vi "main.vi"() -> ()   [LabVIEW 2015]
uses:
  Type Definitions/Tabs.ctl
  Type Definitions/Technique_selector(Combo box).ctl
  Type Definitions/UI_States.ctl
  Type Definitions/UI_Data.ctl
  support VIs/Message Queue/Enqueue Message (Single).vi
  <vilib>/Utility/error.llb/Error Cluster From Error Code.vi
  <vilib>/ErrorRing/Error Ring.xnode
  support VIs/User Event - Stop/User Event - Stop.lvlib
  support VIs/Message Queue/Message Queue.lvlib
  Techniques/CV/CV.lvlib
panel:
  in  "Combo Box":T1
  in  "Tabs":T2
  out "Cluster 2":T3
  in  "Error In":errorcluster
  in  "Preferences Button":bool
  in  "Settings Button":bool
  in  "File Path Control":path
  in  "Play Button":bool
  in  "Record Button":bool
  in  "Process Stop Button":bool
  in  "Stop Button":bool
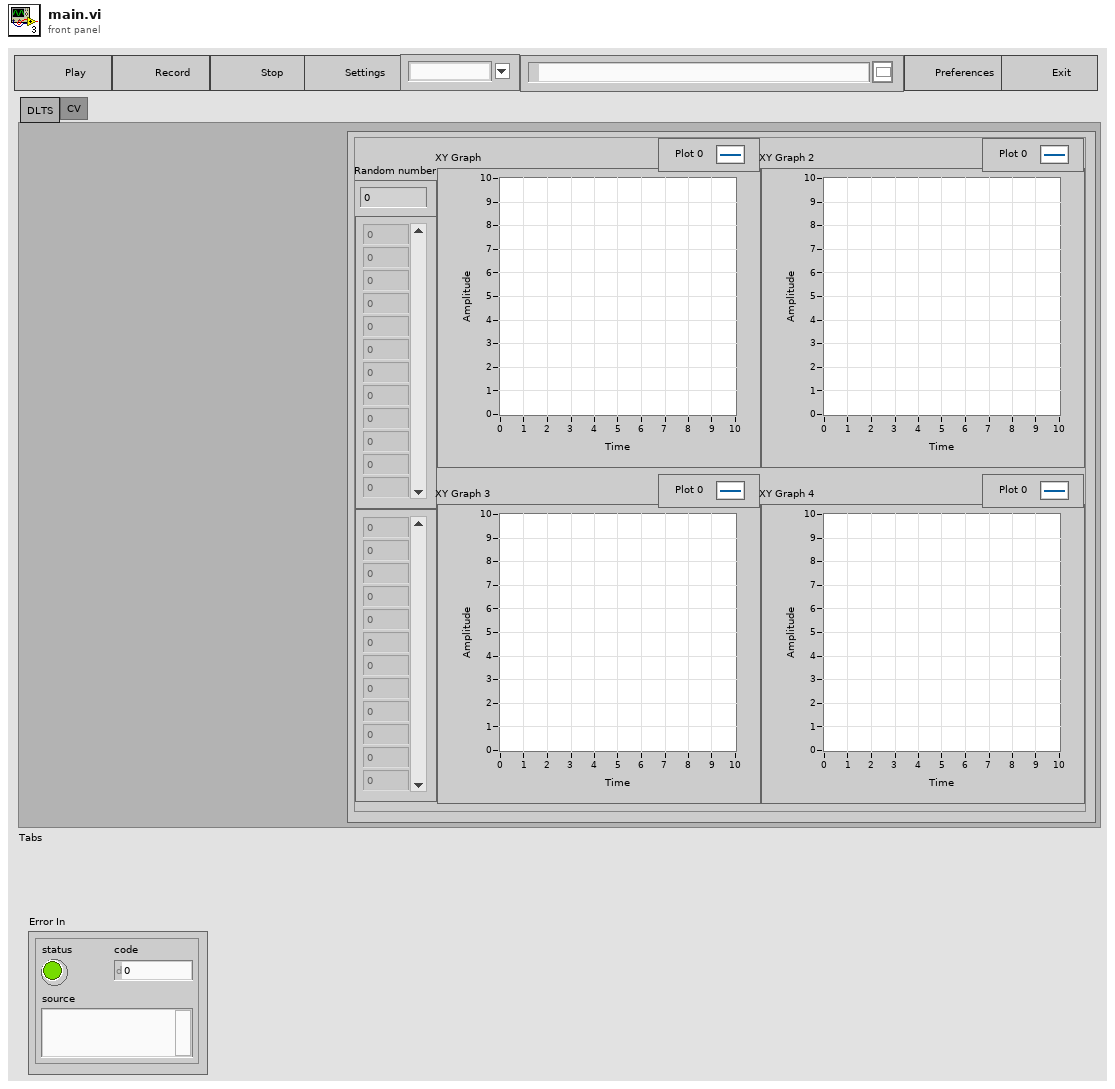
[diagram p1: front panel]
types:
  T1 = typedef "Technique_selector(Combo box).ctl" = string
  T2 = typedef "Tabs.ctl" = enum32{"DLTS", "CV"}
  T3 = cluster{"Array - Numeric 2":dbl[], "XY Graph":cluster{"X":dbl, "Y":dbl}[], "XY Graph 2":cluster{"X":dbl, "Y":dbl}[], "XY Graph 3":cluster{"X":dbl, "Y":dbl}[], "XY Graph 4":cluster{"X":dbl, "Y":dbl}[], "Array - Numeric":dbl[], "Random number":dbl}
  T4 = typedef "UI_Data.ctl" = cluster{"Play Button":refnum<vi>, "Record Button":refnum<vi>, "Stop Button":refnum<vi>, "Settings Button":refnum<vi>, "Preferences Button":refnum<vi>, "Exit Button":refnum<vi>, "Technique Enum":refnum<vi>, "File Path":refnum<vi>}
  T5 = typedef "UI_States.ctl" = enum16{"Idle", "Acquiring and Logging", "Waiting for Exit", "Waiting for Exit (Acq Stoppet)", "Waiting for Exit (Log Stoppet)", "Waiting for Stop", "Waiting for Stop (Acq Stoppet)", "Waiting for Stop (Log Stoppet)"}
  T6 = typedef "Message Queue.lvlib/All Message Queues.ctl" = cluster{"UI":refnum<queue>, "CV Acquisition":refnum<queue>, "CV Logging":refnum<queue>, "IV Acquisition":refnum<queue>, "IV Logging":refnum<queue>, "DLTS Acquisiton":refnum<queue>, "DLTS Logging":refnum<queue>, "Acquisition":refnum<queue>, "Logging":refnum<queue>}
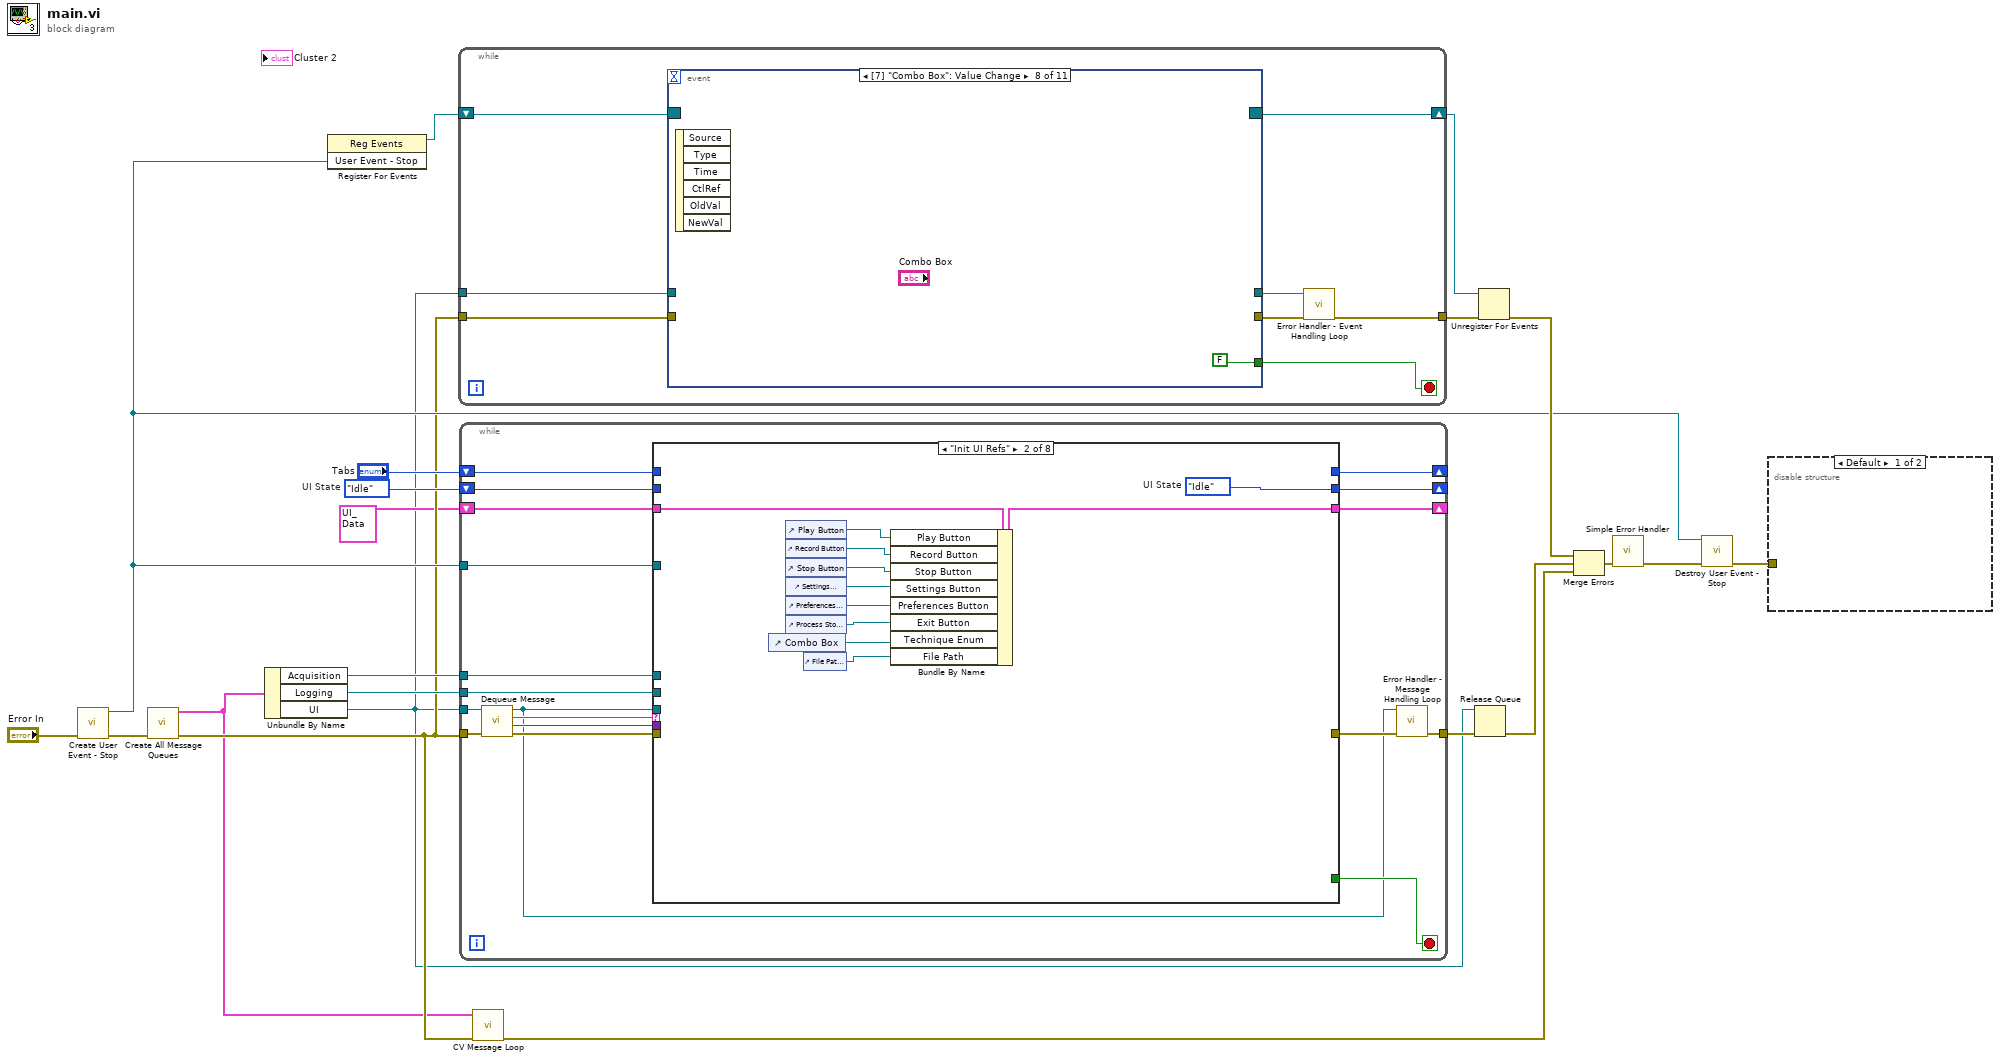
[diagram p0: block diagram]
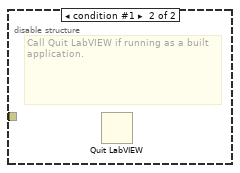
[diagram p2: hidden frame]
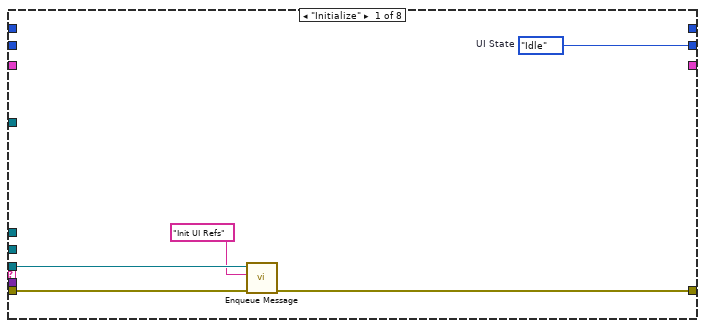
[diagram p3: hidden frame]
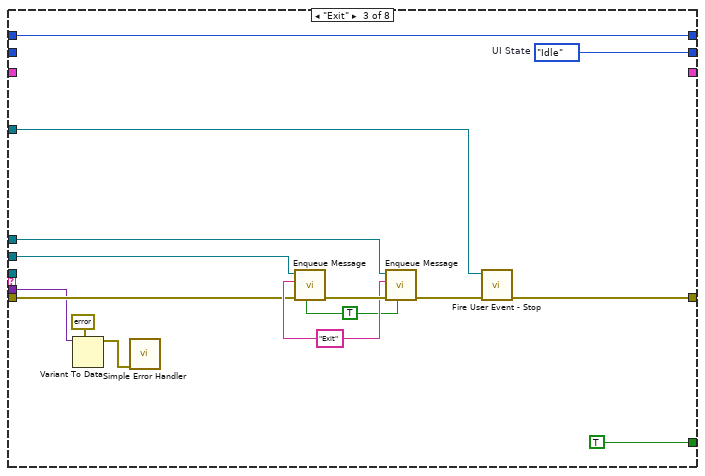
[diagram p4: hidden frame]
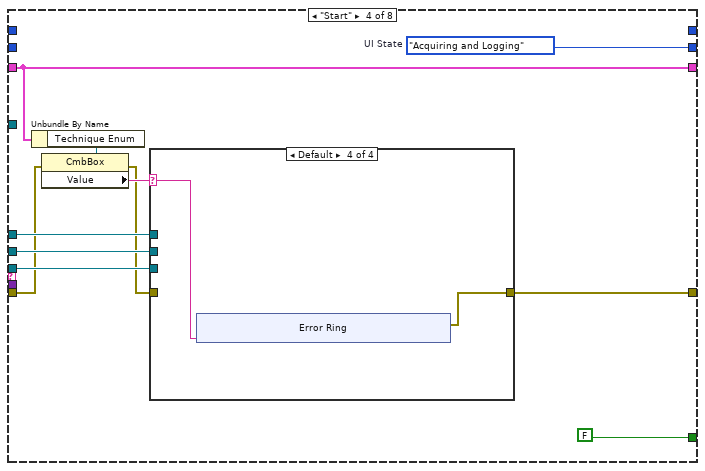
[diagram p5: hidden frame]
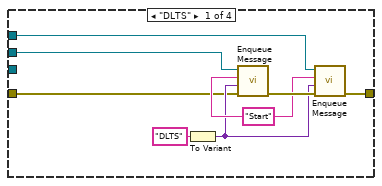
[diagram p6: hidden frame]
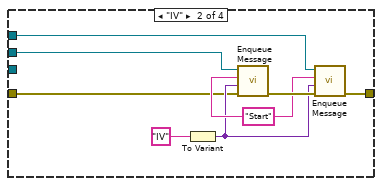
[diagram p7: hidden frame]
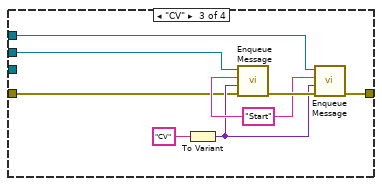
[diagram p8: hidden frame]
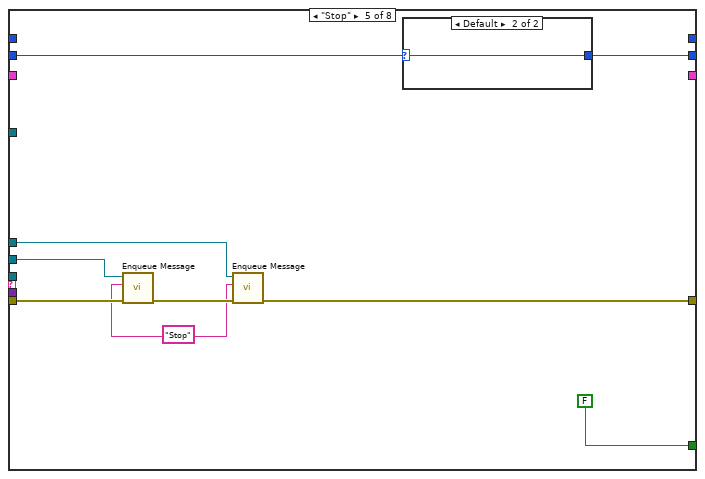
[diagram p9: hidden frame]
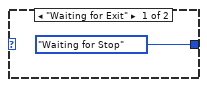
[diagram p10: hidden frame]
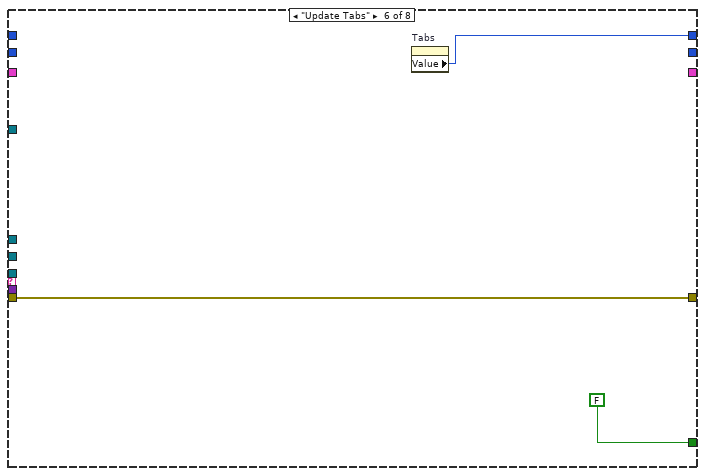
[diagram p11: hidden frame]
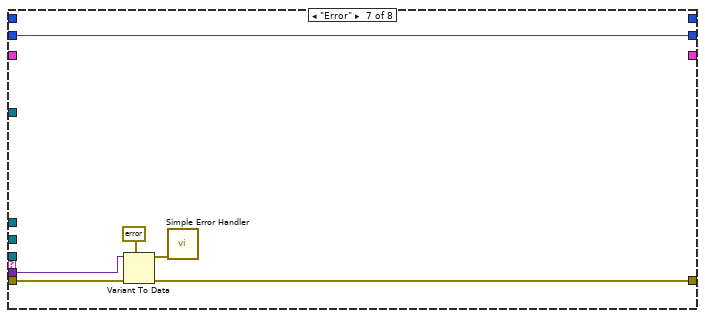
[diagram p12: hidden frame]
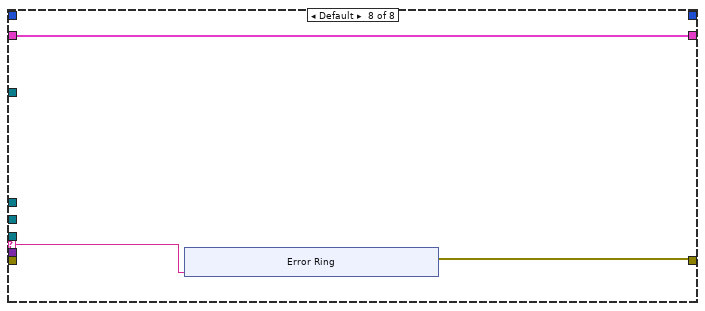
[diagram p13: hidden frame]
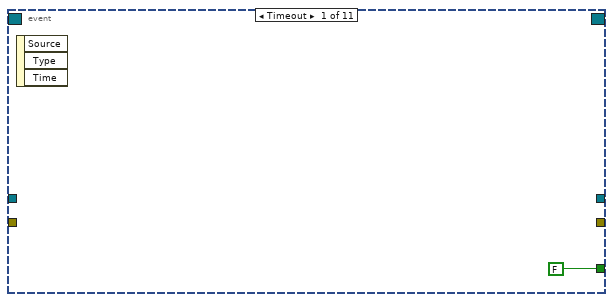
[diagram p14: hidden frame]
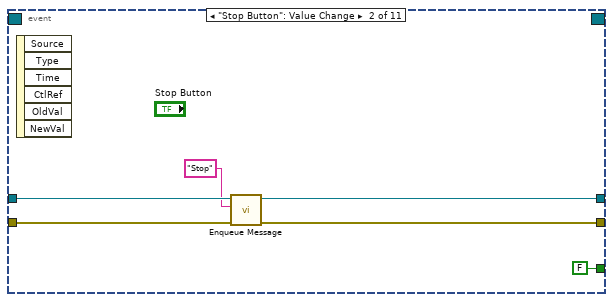
[diagram p15: hidden frame]
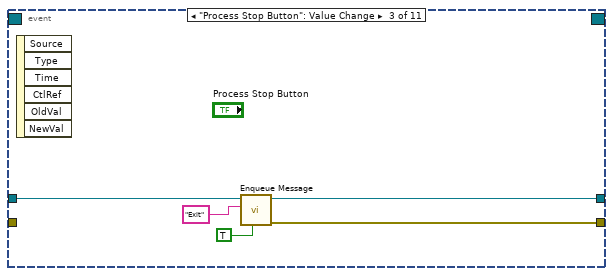
[diagram p16: hidden frame]
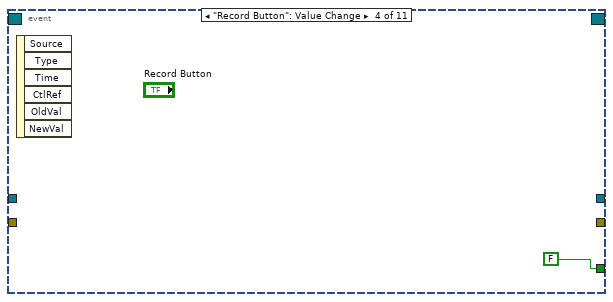
[diagram p17: hidden frame]
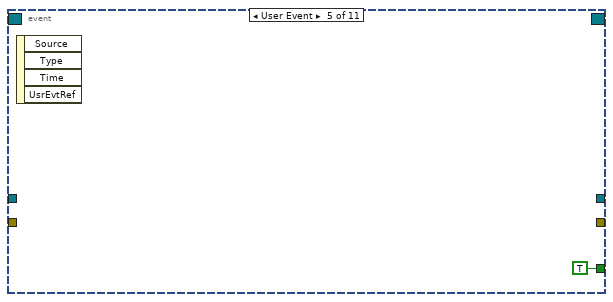
[diagram p18: hidden frame]
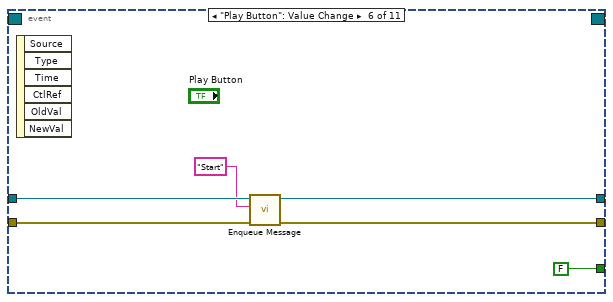
[diagram p19: hidden frame]
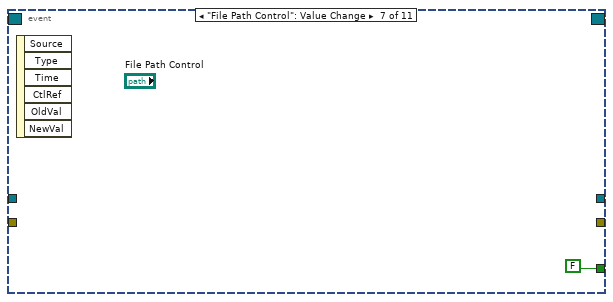
[diagram p20: hidden frame]
diagram:
  w11 = UI_States."Idle"  # UI State
  n1 = call "Create User Event - Stop.vi"("error in (no error)"="Error In") -> ("error out"=w19:errorcluster, "User Event - Stop"=w12:refnum<user-event>)  [unwired: 9 in]
  n2 = call "Create All Message Queues.vi"("error in (no error)"=w19) -> ("error out"=w9:errorcluster, "Message Queues out"=w8:T6)  [unwired: 9 in]
  n3 = Unbundle By Name(w8) -> ("Acquisition"=w10:refnum<queue>, "Logging"=w13:refnum<queue>, "UI"=w2:refnum<queue>)
  n4 = register-events(w12) -> (reference out=w18:refnum<event-registration>)  [unwired: 2 in, 1 out]
  n5 = while {
    shift-right: [w27] -> w16
    shift-left: w18 -> [w28]
    tunnel: w2 -> [w26]
    tunnel: [w23] -> w17
    tunnel: w9 -> [w25]
    stop <- w29 stop-if-true
    n6 = event shown="[7] \"Combo Box\": Value Change" {
      selector: w28 -> [_ _ _ _ _ _ _ _ _ _ _]
      dyn-events: [_ _ _ _ _ _ _ _ _ _ _] -> w27
      timeout: _ -> [_ _ _ _ _ _ _ _ _ _ _]
      tunnel: [FALSE ("Process Stop Button") FALSE ("Process Stop Button") _ FALSE ("Process Stop Button") TRUE ("Process Stop Button") FALSE ("Process Stop Button") FALSE ("Process Stop Button") FALSE ("Process Stop Button") FALSE ("Process Stop Button") FALSE ("Process Stop Button") _] -> w29
      tunnel: w26 -> [_ w34 w41 _ _ w48 _ _ _ _ w56]
      tunnel: [_ w31 w40 _ _ w45 _ _ _ _ w57] -> w22
      tunnel: [_ w32 w39 _ _ w46 _ _ _ _ _] -> w24
      tunnel: w25 -> [_ w35 _ _ _ w47 _ _ _ _ w55]
      event Timeout {
        n7 = event-data() -> ()  [unwired: 1 in, 3 out]
      }
      event "Stop Button": Value Change {
        n8 = event-data() -> ()  [unwired: 1 in, 6 out]
        n9 = call-poly "Enqueue Message.vi"("error in (no error)"=w35, "Message"="Stop", "Message Queue"=w34) -> ("error out"=w32:errorcluster, "dup Message Queue"=w31:refnum<queue>)  [unwired: 7 in]
      }
      event "Process Stop Button": Value Change {
        n10 = event-data() -> ()  [unwired: 1 in, 6 out]
        n11 = call-poly "Enqueue Message.vi"("Priority Message? (F)"=TRUE, "Message"="Exit", "Message Queue"=w41) -> ("error out"=w39:errorcluster, "dup Message Queue"=w40:refnum<queue>)  [unwired: 7 in]
      }
      event "Record Button": Value Change {
        n12 = event-data() -> ()  [unwired: 1 in, 6 out]
      }
      event User Event {
        n13 = event-data() -> ()  [unwired: 1 in, 4 out]
      }
      event "Play Button": Value Change {
        n14 = event-data() -> ()  [unwired: 1 in, 6 out]
        n15 = call-poly "Enqueue Message.vi"("error in (no error)"=w47, "Message"="Start", "Message Queue"=w48) -> ("error out"=w46:errorcluster, "dup Message Queue"=w45:refnum<queue>)  [unwired: 7 in]
      }
      event "File Path Control": Value Change {
        n16 = event-data() -> ()  [unwired: 1 in, 6 out]
      }
      event Value Change {
        n17 = event-data() -> ()  [unwired: 1 in, 6 out]
      }
      event "Settings Button": Value Change {
        n18 = event-data() -> ()  [unwired: 1 in, 6 out]
      }
      event "Preferences Button": Value Change {
        n19 = event-data() -> ()  [unwired: 1 in, 6 out]
      }
      event Value Change {
        n20 = event-data() -> ()  [unwired: 1 in, 6 out]
        n21 = call-poly "Enqueue Message.vi"("error in (no error)"=w55, "Message"="Update Tabs", "Message Queue"=w56) -> ("dup Message Queue"=w57:refnum<queue>)  [unwired: 7 in, 1 out]
      }
    }
    n22 = call "Error Handler - Event Handling Loop.vi"("error in (no error)"=w24, "Message Queue"=w22) -> ("dup error in"=w23:errorcluster)  [unwired: 8 in, 1 out]
  }
  n23 = while {
    tunnel: w2 -> [w75]
    tunnel: w9 -> [w71]
    shift-right: [w68] -> _
    shift-left: "Tabs" -> [w69]
    tunnel: w12 -> [w67]
    tunnel: [w65] -> w3
    tunnel: w13 -> [w66]
    shift-right: [w61] -> _
    shift-left: w11 -> [w62]
    tunnel: w10 -> [w60]
    shift-right: [w58] -> _
    shift-left: T4 {"Play Button"=refnum, "Record Button"=refnum, "Stop Button"=refnum, "Settings Button"=refnum, "Preferences Button"=refnum, "Exit Button"=refnum, "Technique Enum"=refnum, "File Path"=refnum} -> [w59]
    stop <- w70 stop-if-true
    n24 = call "Dequeue Message.vi"("error in (no error)"=w71, "Message Queue"=w75) -> ("error out"=w72:errorcluster, "Message Data"=w73:variant, "Message"=w74:string, "dup Message Queue"=w63:refnum<queue>)  [unwired: 6 in]
    n25 = case shown="\"Init UI Refs\"" w74 {
      selector: w74 -> [_ _ _ _ _ _ _ w172]
      tunnel: w63 -> [w79 _ _ w115 _ _ _ _]
      tunnel: w73 -> [_ _ w94 _ _ _ w168 _]
      tunnel: w72 -> [w80 _ w99 w108 w159 w163 w167 _]
      tunnel: [_ _ TRUE ("true") FALSE ("true") FALSE ("true") FALSE _ _] -> w70
      tunnel: w69 -> [_ _ w106 _ _ _ _ _]
      tunnel: [_ _ w106 _ _ w162 _ _] -> w68
      tunnel: w67 -> [_ _ w105 _ _ _ _ _]
      tunnel: [w78 _ w104 w114 w155 w163 w166 w171] -> w64
      tunnel: w66 -> [_ _ w101 w113 w157 _ _ _]
      tunnel: w62 -> [_ _ _ _ w152 _ w165 _]
      tunnel: [w77 w82 w96 w116 w151 _ w165 _] -> w61
      tunnel: w60 -> [_ _ w98 w112 w153 _ _ _]
      tunnel: w59 -> [_ w91 _ w109 _ _ _ w173]
      tunnel: [_ w90 _ w109 _ _ _ w173] -> w58
      frame "Initialize" {
        w77 = UI_States."Idle"  # UI State
        n26 = call-poly "Enqueue Message.vi"("error in (no error)"=w80, "Message"="Init UI Refs", "Message Queue"=w79) -> ("error out"=w78:errorcluster)  [unwired: 7 in, 1 out]
      }
      frame "Init UI Refs" {
        w82 = UI_States."Idle"  # UI State
        n27 = control-ref of="Combo Box"() -> (w81:refnum<vi>)
        n28 = control-ref of="Play Button"() -> (w89:refnum<vi>)
        n29 = control-ref of="Record Button"() -> (w85:refnum<vi>)
        n30 = control-ref of="Stop Button"() -> (w84:refnum<vi>)
        n31 = control-ref of="Settings Button"() -> (w88:refnum<vi>)
        n32 = control-ref of="Preferences Button"() -> (w87:refnum<vi>)
        n33 = control-ref of="Process Stop Button"() -> (w86:refnum<vi>)
        n34 = control-ref of="File Path Control"() -> (w83:refnum<vi>)
        n35 = Bundle By Name(cluster=w91, "Play Button"=w89, "Record Button"=w85, "Stop Button"=w84, "Settings Button"=w88, "Preferences Button"=w87, "Exit Button"=w86, "Technique Enum"=w81, "File Path"=w83) -> (w90:T4)
      }
      frame "Exit" {
        w96 = UI_States."Idle"  # UI State
        w97 = TRUE
        w100 = "Exit"
        n36 = Variant To Data(type=errorcluster {"status"=FALSE, "code"=0, "source"=""} ("error constant"), Variant=w94) -> (data=w92:errorcluster)  [unwired: 1 in, 1 out]
        n37 = call <vilib>:"Simple Error Handler.vi"("error in (no error)"=w92) -> ()  [unwired: 4 in, 5 out]
        n38 = call-poly "Enqueue Message.vi"("Priority Message? (F)"=w97, "error in (no error)"=w99, "Message"=w100, "Message Queue"=w101) -> ("error out"=w103:errorcluster)  [unwired: 6 in, 1 out]
        n39 = call-poly "Enqueue Message.vi"("Priority Message? (F)"=w97, "error in (no error)"=w103, "Message"=w100, "Message Queue"=w98) -> ("error out"=w102:errorcluster)  [unwired: 6 in, 1 out]
        n40 = call "Fire User Event - Stop.vi"("error in (no error)"=w102, "User Event - Stop"=w105) -> ("error out"=w104:errorcluster)  [unwired: 9 in]
      }
      frame "Start" {
        w116 = UI_States."Acquiring and Logging"  # UI State
        n41 = Unbundle By Name(w109) -> ("Technique Enum"=w111:refnum<vi>)
        n42 = property class="CmbBox"(reference=w111, error in=w108) -> (error out=w107:errorcluster, "Value"=w110:string)  [unwired: 1 out]
        n43 = case shown="Default" w110 {
          selector: w110 -> [_ _ _ w142]
          tunnel: w107 -> [w118 w126 w134 _]
          tunnel: w115 -> [_ _ _ _]
          tunnel: [w124 w132 w140 w143] -> w114
          tunnel: w113 -> [w123 w131 w139 _]
          tunnel: w112 -> [w122 w130 w138 _]
          frame "DLTS" {
            w121 = "Start" ("Message")
            n44 = To Variant(anything="DLTS") -> (Variant=w119:variant)
            n45 = call-poly "Enqueue Message.vi"("error in (no error)"=w118, "Message Data"=w119, "Message"=w121, "Message Queue"=w123) -> ("error out"=w125:errorcluster)  [unwired: 6 in, 1 out]
            n46 = call-poly "Enqueue Message.vi"("error in (no error)"=w125, "Message Data"=w119, "Message"=w121, "Message Queue"=w122) -> ("error out"=w124:errorcluster)  [unwired: 6 in, 1 out]
          }
          frame "IV" {
            w129 = "Start" ("Message")
            n47 = To Variant(anything="IV") -> (Variant=w127:variant)
            n48 = call-poly "Enqueue Message.vi"("error in (no error)"=w126, "Message Data"=w127, "Message"=w129, "Message Queue"=w131) -> ("error out"=w133:errorcluster)  [unwired: 6 in, 1 out]
            n49 = call-poly "Enqueue Message.vi"("error in (no error)"=w133, "Message Data"=w127, "Message"=w129, "Message Queue"=w130) -> ("error out"=w132:errorcluster)  [unwired: 6 in, 1 out]
          }
          frame "CV" {
            w137 = "Start" ("Message")
            n50 = To Variant(anything="CV") -> (Variant=w135:variant)
            n51 = call-poly "Enqueue Message.vi"("error in (no error)"=w134, "Message Data"=w135, "Message"=w137, "Message Queue"=w139) -> ("error out"=w141:errorcluster)  [unwired: 6 in, 1 out]
            n52 = call-poly "Enqueue Message.vi"("error in (no error)"=w141, "Message Data"=w135, "Message"=w137, "Message Queue"=w138) -> ("error out"=w140:errorcluster)  [unwired: 6 in, 1 out]
          }
          frame Default {
            n53 = xnode "Error Ring"("parameter 0"=w142) -> ("error out"=w143:errorcluster)
          }
        }
      }
      frame "Stop" {
        w154 = "Stop" ("Message")
        n54 = call-poly "Enqueue Message.vi"("error in (no error)"=w159, "Message"=w154, "Message Queue"=w157) -> ("error out"=w156:errorcluster)  [unwired: 7 in, 1 out]
        n55 = call-poly "Enqueue Message.vi"("error in (no error)"=w156, "Message"=w154, "Message Queue"=w153) -> ("error out"=w155:errorcluster)  [unwired: 7 in, 1 out]
        n56 = case shown="Default" w152 {
          selector: w152 -> [_ w161]
          tunnel: [UI_States."Waiting for Stop" ("UI State") w161] -> w151
          frame "Waiting for Exit" {
          }
          frame Default {
          }
        }
      }
      frame "Update Tabs" {
        n57 = property on="Tabs" class="TabCtl (strict)"() -> ("Value"=w162:T2)  [unwired: 2 in, 2 out]
      }
      frame "Error" {
        n58 = Variant To Data(error in=w167, type=errorcluster {"status"=FALSE, "code"=0, "source"=""} ("error constant"), Variant=w168) -> (data=w169:errorcluster, error out=w166:errorcluster)
        n59 = call <vilib>:"Simple Error Handler.vi"("error in (no error)"=w169) -> ()  [unwired: 4 in, 5 out]
      }
      frame Default {
        n60 = xnode "Error Ring"("parameter 0"=w172) -> ("error out"=w171:errorcluster)
      }
    }
    n61 = call "Error Handler - Message Handling Loop.vi"("error in (no error)"=w64, "Message Queue"=w63) -> ("dup error in"=w65:errorcluster)  [unwired: 8 in, 1 out]
  }
  n62 = call "CV Message Loop.vi"("Error In"=w9, "Message Queues"=w8) -> ("Error Out"=w7:errorcluster)  [unwired: 9 in]
  n63 = Release Queue(queue=w2, error in (no error)=w3) -> (error out=w1:errorcluster)  [unwired: 1 in, 2 out]
  n64 = Unregister For Events(event registration refnum=w16, error in=w17) -> (error out=w14:errorcluster)
  n65 = Merge Errors(w14, w1, w7) -> (w6:errorcluster)
  n66 = call <vilib>:"Simple Error Handler.vi"("error in (no error)"=w6) -> ("error out"=w5:errorcluster)  [unwired: 4 in, 4 out]
  n67 = call "Destroy User Event - Stop.vi"("error in (no error)"=w5, "User Event - Stop"=w12) -> ("error out"=w20:errorcluster)  [unwired: 9 in]
  n68 = disable-structure shown="Default" {
    disable-tunnel: w20 -> [_ _]
    frame condition #0 (active) {
    }
    frame condition #1 {
      # "Call Quit LabVIEW if running as a built application."
      n69 = Quit LabVIEW() -> ()  [unwired: 1 in]
    }
  }
